vi "coerceAngularCoef.vi"(0 "object in":refnum<class "DefendGoalTactic.lvclass">, 1 "Coef ang":dbl, 2 "Field":refnum<class "Field.lvclass">, 3 "Ball":refnum<class "Ball.lvclass">, 5 "error in (no error)":errorcluster) -> (14 "object out":refnum<class "DefendGoalTactic.lvclass">, 17 "coerced(x)":dbl, 19 "error out":errorcluster)   [LabVIEW 2024, in "DefendGoalTactic.lvclass"]
uses:
  DefendGoalTactic.lvclass
  Field_class/Field.lvclass
  Ball_class/Ball.lvclass
  C:/Users/ROBOIME2/Documents/SSL ROBOIME/SSL_AI/Object_class/Object.lvclass
  Object_class/Object.lvclass/Object.ctl
  Field_class/Field.lvclass/Field.ctl
  Object_class/Read position(x,y).vi
  Field_class/Read ourGoalPosition.vi
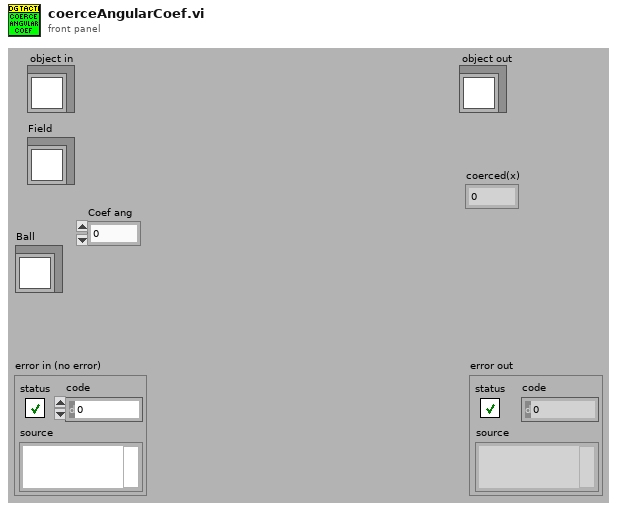
[diagram p1: front panel]
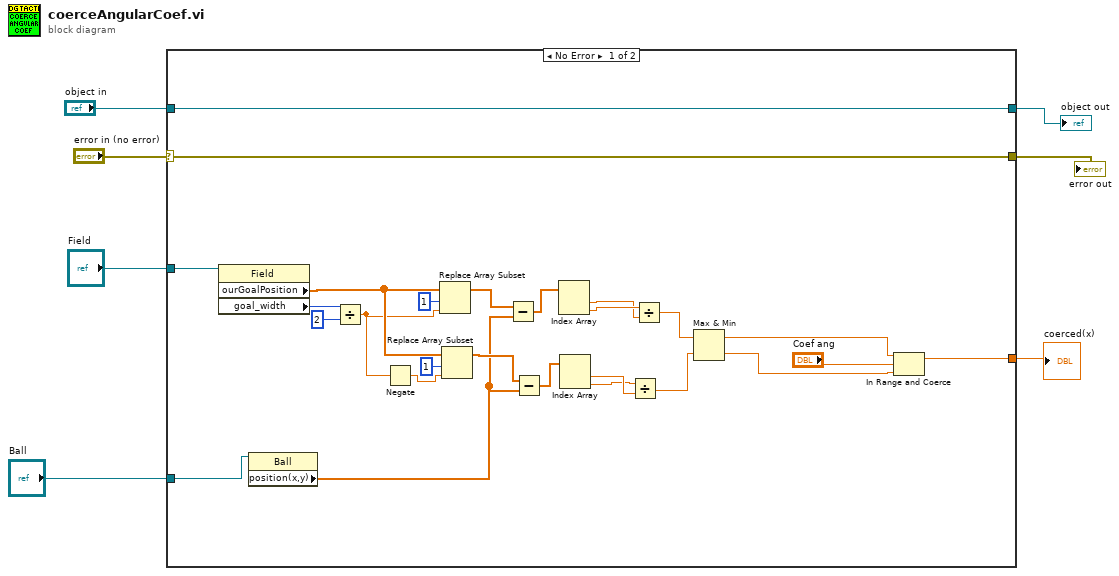
[diagram p0: block diagram]
diagram:
  n1 = case shown="No Error" "error in (no error)" {
    selector: "error in (no error)" -> [w32 w35]
    tunnel: [w32 w35] -> w6
    tunnel: [w33 w34] -> w4
    tunnel: "object in" -> [w33 w34]
    tunnel: "Field" -> [w31 _]
    tunnel: "Ball" -> [w30 _]
    tunnel: [w8 _] -> w1
    frame No Error {
      n2 = property class="Field"(reference=w31) -> ("ourGoalPosition"=w29:dbl[], "goal_width"=w26:i32)  [unwired: 1 in, 2 out]
      n3 = property class="Ball"(reference=w30) -> ("position(x,y)"=w12:dbl[])  [unwired: 1 in, 2 out]
      n4 = Divide(x=w26, y=2) -> (x/y=w24:dbl)
      n5 = Negate(x=w24) -> (-x=w23:dbl)
      n6 = Replace Array Subset(array=w29, new element=w24, index=1) -> (w11:dbl[])
      n7 = Replace Array Subset(array=w29, new element=w23, index=1) -> (w13:dbl[])
      n8 = Subtract(x=w11, y=w12) -> (x-y=w9:dbl[])
      n9 = Subtract(x=w13, y=w12) -> (x-y=w10:dbl[])
      n10 = Index Array(array=w9) -> (element #1=w19:dbl, element #2=w20:dbl)  [unwired: 2 in]
      n11 = Index Array(array=w10) -> (element #1=w22:dbl, element #2=w21:dbl)  [unwired: 2 in]
      n12 = Divide(x=w21, y=w22) -> (x/y=w16:dbl)
      n13 = Divide(x=w20, y=w19) -> (x/y=w17:dbl)
      n14 = Max & Min(x=w17, y=w16) -> (max(x,y)=w15:dbl, min(x,y)=w14:dbl)
      n15 = In Range and Coerce(upper limit=w15, x="Coef ang", lower limit=w14) -> (coerced(x)=w8:dbl)  [unwired: 1 out]
    }
    frame Error {
    }
  }
  "error out" <- w6
  "object out" <- w4
  "coerced(x)" <- w1
